vi "Slave Init.vi"(8 "error in (no error)":errorcluster, 9 "ID":i32, 11 "Master in":refnum<class "Master.lvclass">) -> (0 "error out":errorcluster, 3 "Master out":refnum<class "Master.lvclass">)   [LabVIEW 2021, in "Master.lvlib" / "Master.lvclass"]
uses:
  Master.lvclass
  Master.lvclass/Master.ctl
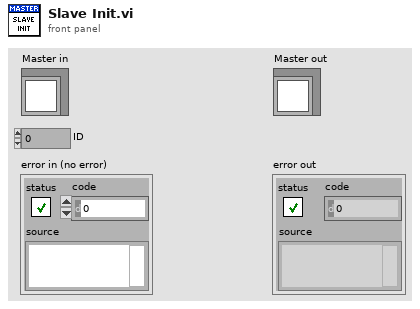
[diagram p1: front panel]
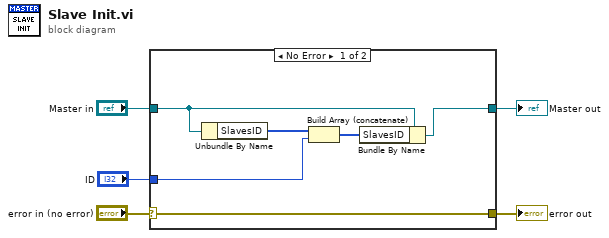
[diagram p0: block diagram]
diagram:
  n1 = case shown="No Error" "error in (no error)" {
    selector: "error in (no error)" -> [w11 w13]
    tunnel: [w11 w13] -> w4
    tunnel: [w6 w12] -> w2
    tunnel: "Master in" -> [w7 w12]
    tunnel: "ID" -> [w8 _]
    frame No Error {
      n2 = Unbundle By Name(w7) -> ("SlavesID"=w9:i32[])
      n3 = Build Array (concatenate)(w9, w8) -> (w10:i32[])
      n4 = Bundle By Name(cluster=w7, "SlavesID"=w10) -> (w6:refnum<class "Master.lvclass">)
    }
    frame Error {
    }
  }
  "error out" <- w4
  "Master out" <- w2
